vi "GUI_kHz_LPA_backup20250620.vi"() -> ()   [LabVIEW 2020]
uses:
  GUI_TestStand/Fire button.ctl
  Shared/GUI_Template/GUI_master/tcp_new_data_event.ctl
  Shared/GUI_Template/GUI_master/tcp new data cluster.ctl
  Device Drivers/DG645/subVIs/TriggerSource_TypDef.ctl
  <vilib>/Utility/config.llb/Write Key (I32).vi
  <vilib>/Utility/config.llb/NI_LVConfig.lvlib
panel:
  in  "BASE PATH":path=path "Z:/software/control-all-loasis/kHzLPA/Active Version"
  in  "stop":bool
  in  "Tab Control":enum32{"Devices", "Parameters", "Shortcuts"}(tab)=enum."Parameters"
  in  "GUIdevice 6":string="FireContinues"
  in  "GUIdevice 2":string="kHz_1Wire"
  in  "GUIdevice 1":string="kHz_Alicat"
  in  "GUIdevice 3":string="kHz_Hexapod_Target"
  in  "GUIdevice 4":string="kHz_DG645_ShotControl"
  in  "GUIdevice 5":string="kHz_Zaber_Compressor"
  out "error IO":errorcluster
  out "tcp data event":T1
  in  "GUIdevice 7":string="kHz_ESP_TC"
  in  "Scan":T2(ring)
  in  "LogTable":bool
  in  "Mode Imager Button":bool caption="Mode Imager In"
  in  "Step size":dbl=0.01 min=0.001 max=1.0 step=0.001 format="%.3f"
  in  "Rate (Hz)":dbl=0.3
  in  "Fire Continues Checkbox":bool
  out "Fire continues Indicator":bool caption="Fire continuous"
  in  "Trigger.Source::4":T3 caption="SRS Trigger Mode"
  in  "<command>::3":bool caption="ABORT"
  in  "Position.Ch1::5":i32 caption="Ch1" min=0 max=250000 step=1
  in  "Position.Channel 1::2":T4(ring) caption="Fiber Mode"
  in  "Position.Channel 2::2":T4(ring) caption="XH2"
  in  "Position.Channel 3::2":T4(ring) caption="ND6"
  in  "Position.Channel 4::2":T4(ring) caption="XH4"
  in  "Position.Channel 5::2":T4(ring) caption="d-scan wedge"
  in  "Position.Channel 6::2":T4(ring) caption="EC wedge"
  in  "Position.Channel 8::2":T4(ring) caption="Gentec"
  in  "Position.Channel 7::2":T4(ring) caption="Pointing Lanex"
  in  "Pressure.device 1::1":dbl=14.0 caption="Target Pressure" min=0.0 max=100.0
  in  "Pressure.device 2::1":dbl=0.1 caption="Fiber Pressure" min=-14.7 max=500.0
  in  "xpos::3":dbl=-18.95 caption="x" min=-22.5 max=22.5 step=0.009999999999999998 format="%.3f"
  in  "zpos::3":dbl=-0.7 caption="z" min=-10.0 max=10.0 step=0.009999999999999998 format="%.3f"
  in  "ypos::3":dbl=10.7 caption="y" min=-22.5 max=22.5 step=0.009999999999999998 format="%.3f"
  in  "uangle::3":dbl caption="u" min=-7.5 max=7.5 step=0.009999999999999998 format="%.3f"
  in  "vangle::3":dbl=0.0007 caption="v" min=-7.5 max=7.5 step=0.009999999999999998 format="%.3f"
  in  "wangle::3":dbl=-0.0001 caption="w" min=-7.5 max=7.5 step=0.009999999999999998 format="%.3f"
  in  "Fire Button":T5=TRUE
  in  "Jet trigger":bool caption="Jet Trigger"
  in  "Jet enable":bool caption="Jet Enable"
  in  "Set opening time (s)":dbl=0.004
  in  "Amplitude.Ch AB::4":dbl=4.0 caption="Amplitude Jet trigger" min=0.5 max=5.0 format="%.1f"
  in  "Delay.Ch B::4":dbl=0.004 caption="Opening time" min=-0.1 max=0.1 format="%#_6p"
  in  "value0:6":bool caption="Fire continues"
  in  "UDP error message":string
  in  "Position.Axis 2::7":dbl caption="Magent Postition" min=-65.0 max=30.0 format="%.2f"
  in  "Position.Axis 1::7":dbl caption="Mode Imager Position" min=0.0 max=25.0 format="%.2f"
  in  "fire::4":string="fire>>force" caption="fire text"
  in  "Position.Axis 3::7":dbl caption="Probe Delay" min=0.0 max=25.0 format="%.2f"
  in  "Create Log":bool caption="LogTable"
  in  "LogEpilog":bool caption="LogTable"
  in  "Gen new log?":bool
  in  "Search Log":bool caption="PicoL GUI"
  in  "RemoteDesktop":bool caption="PicoL GUI"
  in  "kHz Interactive":bool caption="PicoL GUI"
  in  "Exp Editor":bool caption="PicoL GUI"
  in  "DB Editor":bool caption="PicoL GUI"
  in  "AddColumns":bool caption="PicoL GUI"
  in  "GEECSplot":bool caption="PicoL GUI"
  in  "MasterControl":bool caption="PicoL GUI"
  in  "Google Drive":bool
  in  "LVStarter":bool caption="PicoL GUI"
  out "standard output":string="04-16-21\r\n04-16-21 kHz Scanlog\r\nZ:/data/kHzLPA/Y2021/04-Apr/21_0416/scans\\Scan001\r\nSearch updated: 04-16-21.*Scan 1:\r\n**Establish Server Connection with Google Cloud**\r\n...Service created successfully\r\n<googleapiclient.discovery.Resource object at 0x000001F266DE75B0>\r\n**Append template to document...**\r\n... success\r\n**Scanfiles found**\r\nZ:/data/kHzLPA/Y2021/04-Apr/21_0416/ECS Live dumps\\Scan1.txt\r\nZ:/data/kHzLPA/Y2021/04-Apr/21_0416/scans\\Scan001\\ScanInfoScan001.ini\r\n**Find and replace placeholders with current values**\r\n**Establish Server Connection with Google Cloud**\r\n...Service created successfully\r\n<googleapiclient.discovery.Resource object at 0x000001F266EB5790>\r\n**Adding screenshot**\r\n"
  # "kHz control center"
  # "Laser"
  # "1-wire flippers"
  # "\"+x\" is towards laser table\n\"+y\" is towards OAP\n\"+z\" is up"
  # "ABORT !"
  # "Tobi's LogMaker"
  # "Compressor"
  # "Alicat"
  # "New\nScan\nTable"
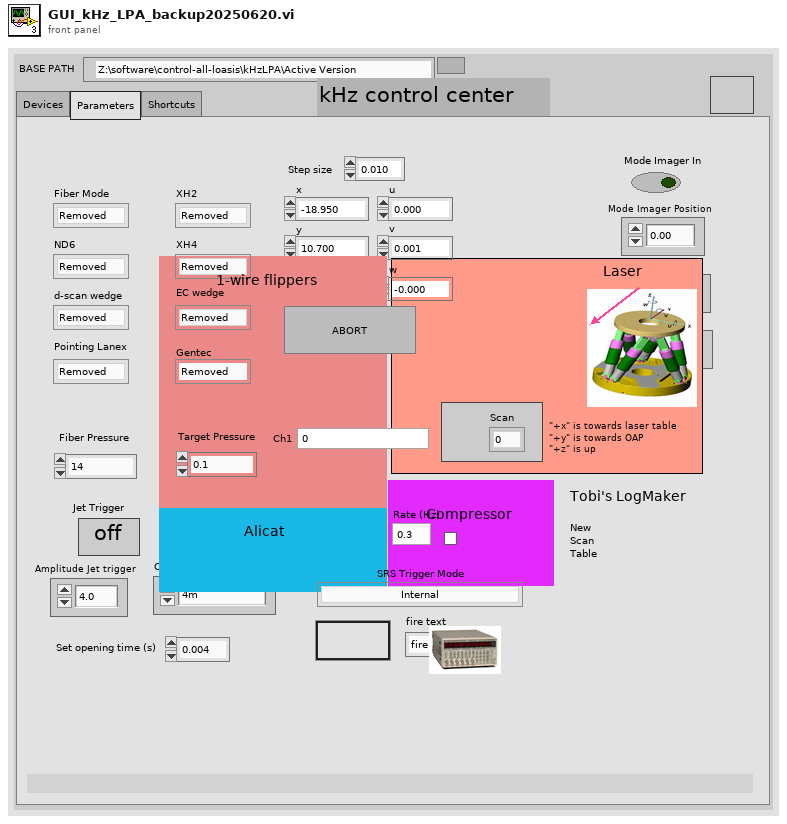
[diagram p1: front panel]
types:
  T1 = typedef "tcp_new_data_event.ctl" = refnum<user-event>
  T2 = enum16{"0", "1", "2", "3", "4", "5", "6", "7", "8", "9", "10", "11", "12", "13", "14", "15", "16", "17", "18", "19", "20", "21", "22", "23", "24", "25", "26", "27", "28", "29", "30", "31", "32", "33", "34", "35", "36", "37", "38", "39", "40", "41", "42", "43", "44", "45", "46", "47", "48", "49", "50", "51", "52", "53", "54", "55", "56", "57", "58", "59", "60", "61", "62", "63", "64", "65", "66", "67", "68", "69", "70", "71", "72", "73", "74", "75", "76", "77", "78", "79", "81", "82", "83", "84", "85", "86", "87", "88", "89", "90", "91", "92", "93", "94", "95", "96", "97", "98", "99", ""}
  T3 = typedef "TriggerSource_TypDef.ctl" = enum16{"Internal", "External rising edges", "External falling edges", "Single shot external rising edges", "Single shot external falling edges", "Single shot", "Line"}
  T4 = enum16{"Removed", "Inserted", "Unknown", "Moving"}
  T5 = typedef "Fire button.ctl" = bool
  T6 = typedef "tcp new data cluster.ctl" = cluster{"EventEnum":enum16{"new data", "connection status update"}, "Device name":string}
  T7 = enum32{"Invalid", "Standard", "Closed", "Hidden", "Minimized", "Maximized"}
  T8 = enum32{"invalid app kind", "Development System", "Run Time System", "Student Edition", "Embedded LabVIEW", "Evaluation", "Custom"}
  T9 = cluster{"Core":cluster{"Current VI Reference":refnum<vi>, "Close Panel on Exit?":bool}, "Jet enable":bool, "Jet trigger":bool, "Fire Continues Allowed":bool, "Tik1":u32, "ModeImagerIn":bool}
  T10 = typedef "imagedata.ctl" = cluster{"image type":i32, "image depth":i32, "image":u8[], "mask":u8[], "colors":u32[], "Rectangle":cluster{"left":i16, "top":i16, "right":i16, "bottom":i16}}
  T11 = typedef "NI_LVConfig.lvlib/Config Data RefNum.ctl" = refnum<k1>
  T12 = cluster{"Current VI Reference":refnum<vi>, "Close Panel on Exit?":bool}
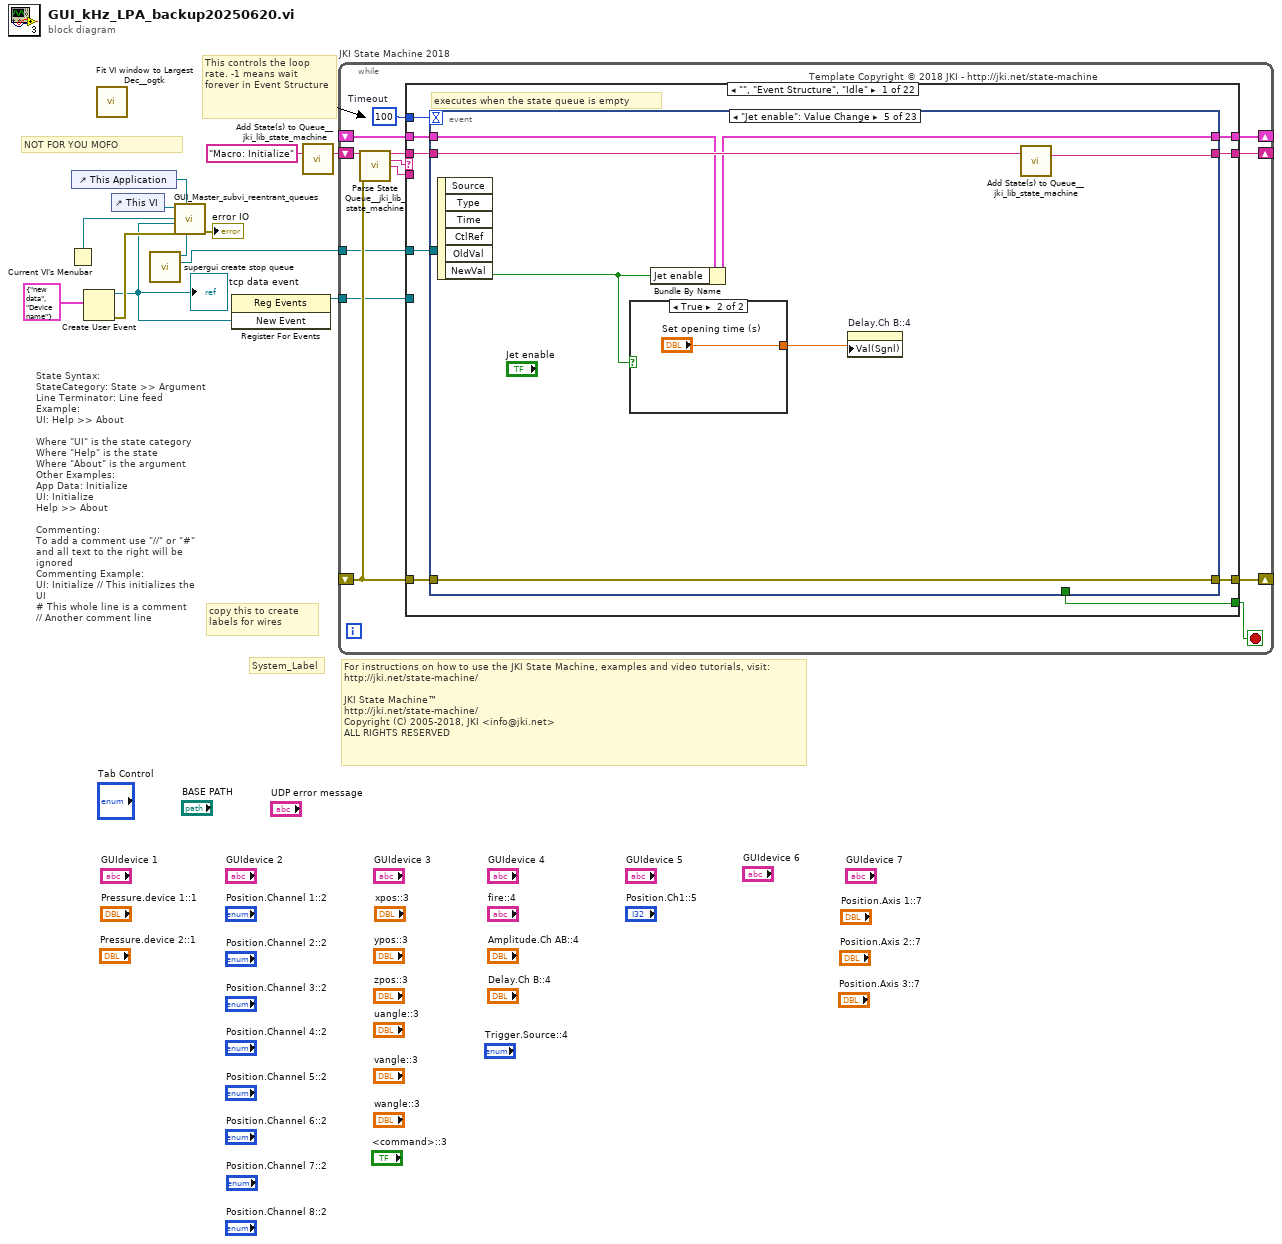
[diagram p0: block diagram]
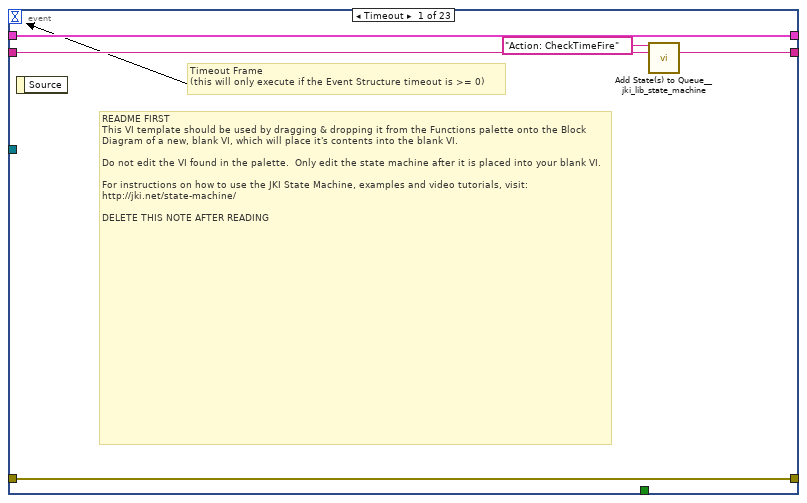
[diagram p2: hidden frame]
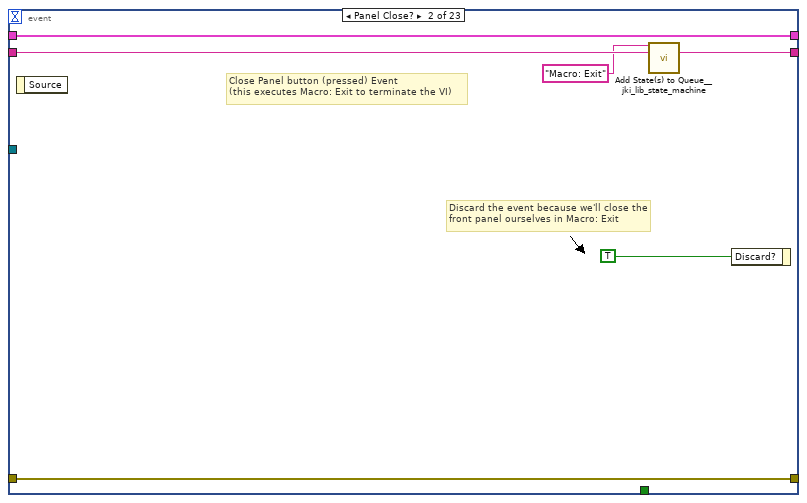
[diagram p3: hidden frame]
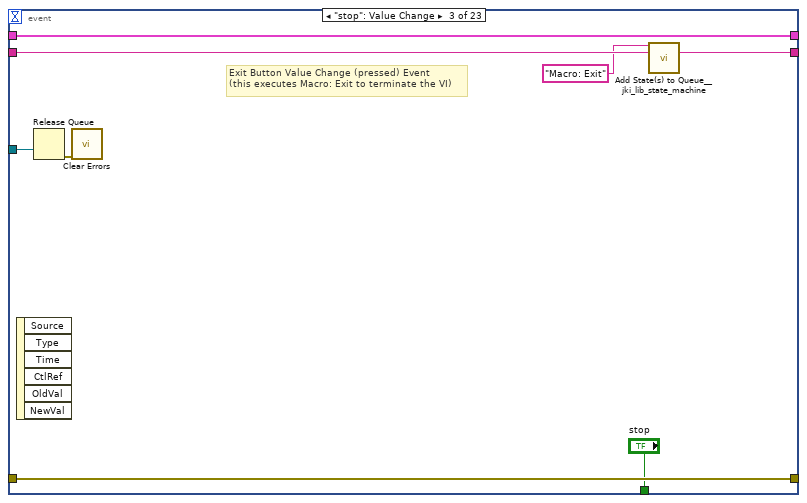
[diagram p4: hidden frame]
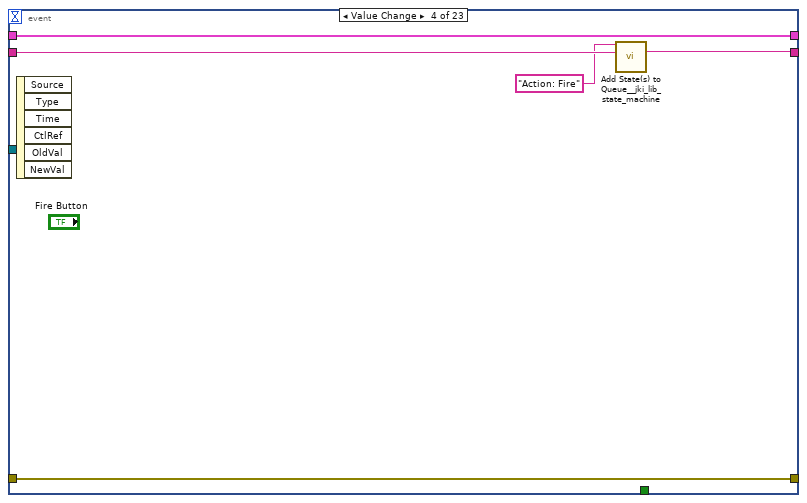
[diagram p5: hidden frame]
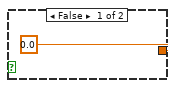
[diagram p6: hidden frame]
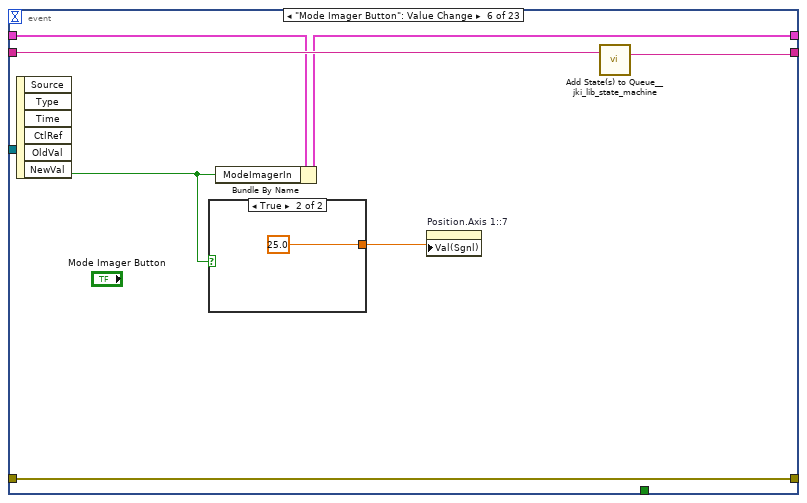
[diagram p7: hidden frame]
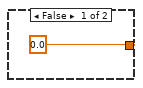
[diagram p8: hidden frame]
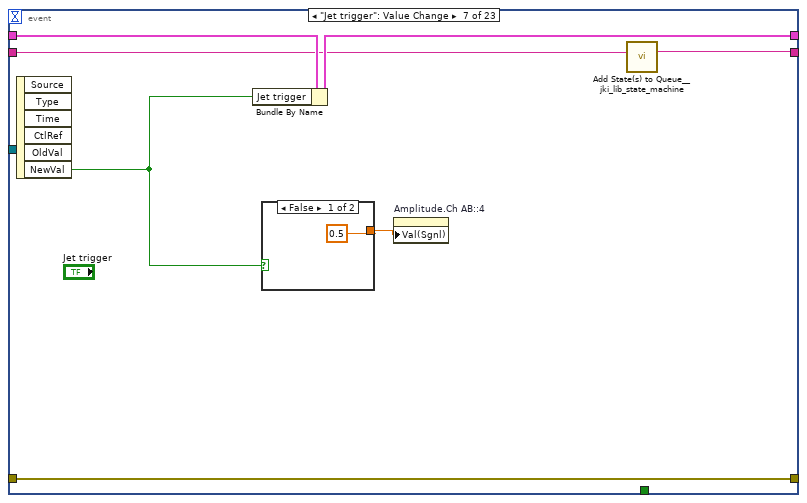
[diagram p9: hidden frame]
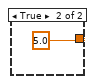
[diagram p10: hidden frame]
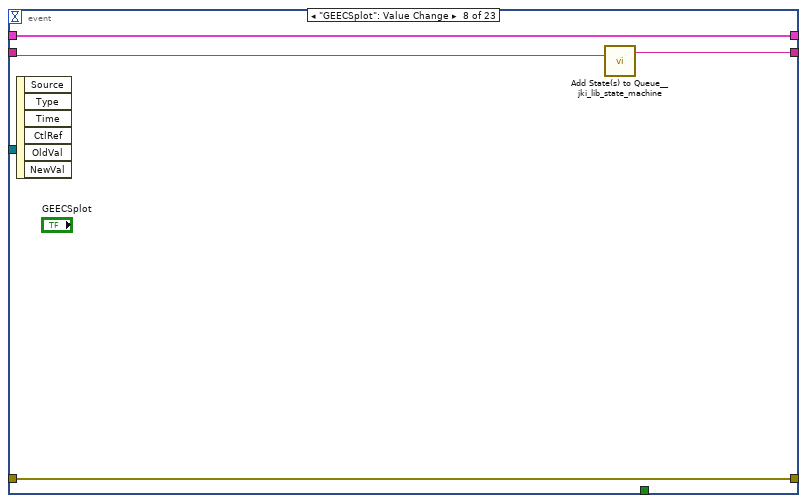
[diagram p11: hidden frame]
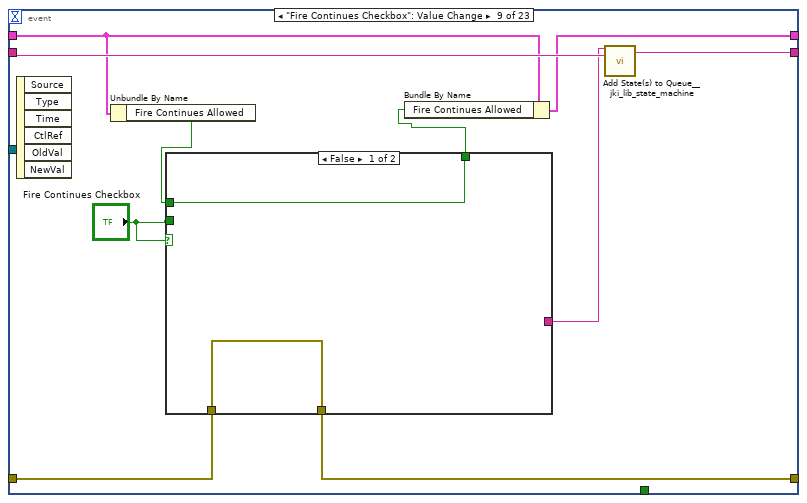
[diagram p12: hidden frame]
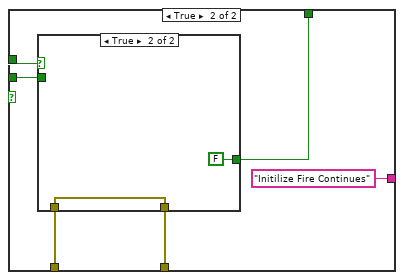
[diagram p13: hidden frame]
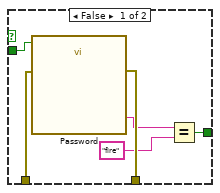
[diagram p14: hidden frame]
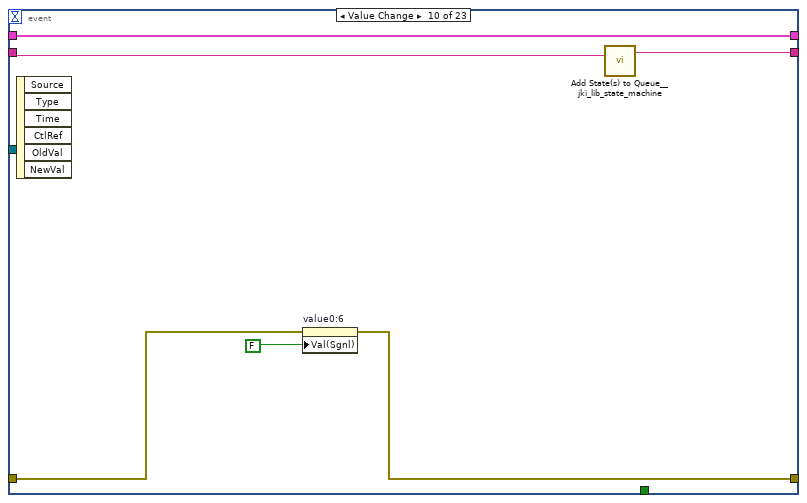
[diagram p15: hidden frame]
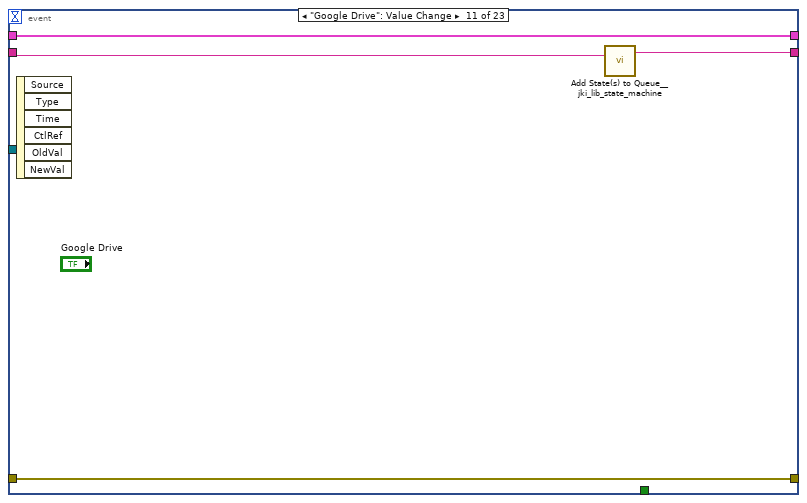
[diagram p16: hidden frame]
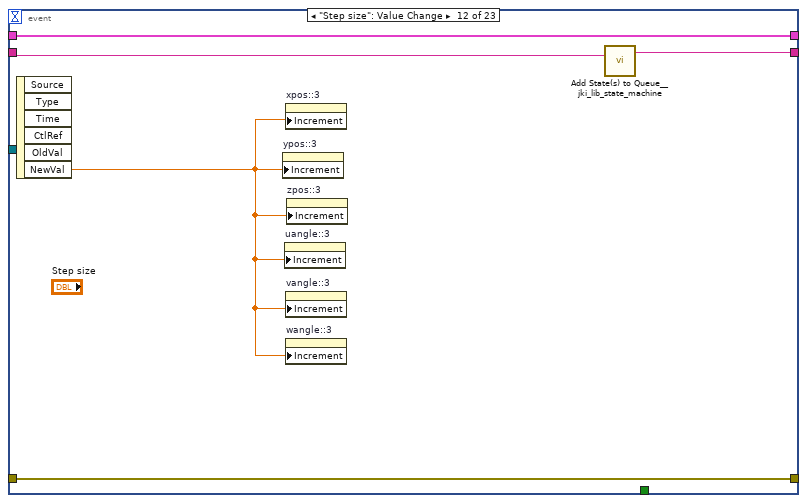
[diagram p17: hidden frame]
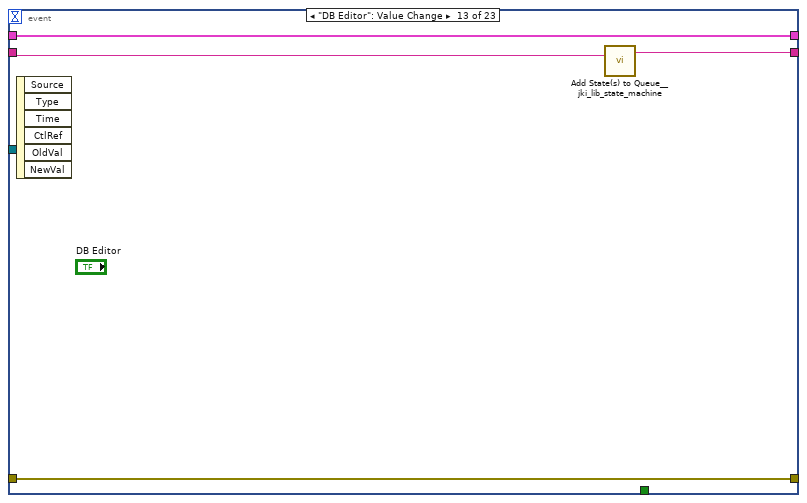
[diagram p18: hidden frame]
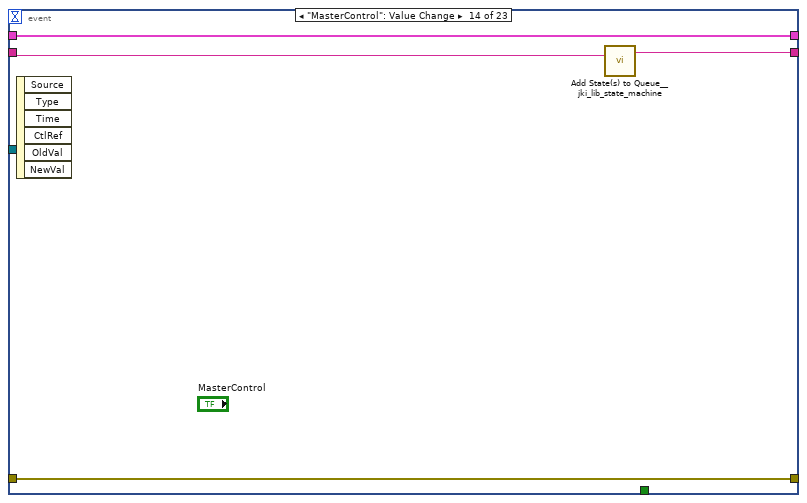
[diagram p19: hidden frame]
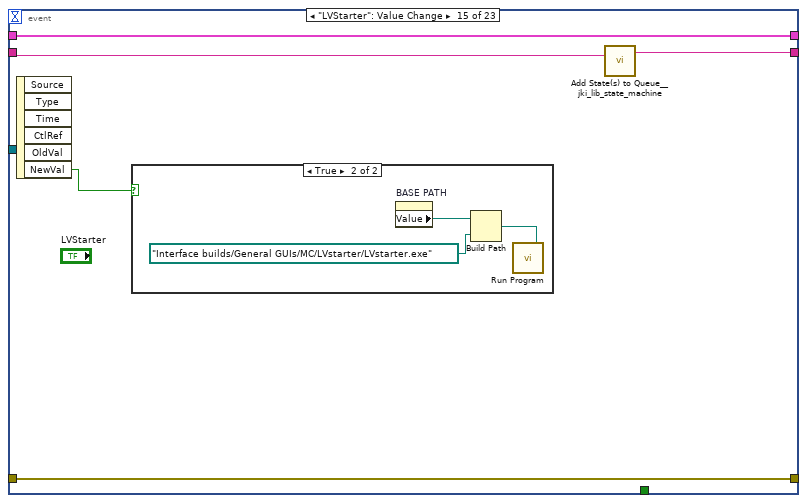
[diagram p20: hidden frame]
diagram:
  # "NOT FOR YOU MOFO"
  # "For instructions on how to use the JKI State Machine, examples and video tutorials, visit:\nhttp://jki.net/state-machine/\n\nJKI State Machine™\nhttp://jki.net/state-machine/\nCopyright (C) 2005-2018, JKI <info@jki.net>\nALL RIGHTS RESERVED"
  # "State Syntax:\nStateCategory: State >> Argument\nLine Terminator: Line feed\nExample:\nUI: Help >> About\n\nWhere \"UI\" is the state category\nWhere \"Help\" is the state\nWhere \"About\" is the argument\nOther Examples:\nApp Data: Initialize\nUI: Initialize\nHelp >> About\n\nCommenting:\nTo add a comment use \"//\" or \"#\" and all text to the right will be ignored\nCommenting Example:\nUI: Initialize // This initializes the UI\n# This whole line is a comment\n// Another comment line"
  # "copy this to create labels for wires"
  # "This controls the loop rate. -1 means wait forever in Event Structure"
  # "System_Label"
  n1 = Current VI's Menubar() -> (w6:refnum<k9>)
  n2 = control-ref of="This Application"() -> (w9:refnum<vi>)
  n3 = Create User Event(user event datatype=T6 {"EventEnum"=enum."new data", "Device name"="Device name"} ("New Event")) -> (user event=w3:refnum<user-event>, error out=w8:errorcluster)  [unwired: 1 in]
  "tcp data event" <- w3
  n4 = call <userlib>:"Fit VI window to Largest Dec__ogtk.vi"() -> ()  [unwired: 6 in, 2 out]
  n5 = control-ref of="This VI"() -> (w5:refnum<vi>)
  n6 = call "supergui create stop queue.vi"() -> ("STOP Queue out"=w2:refnum<queue>)  [unwired: 11 in]
  n7 = call "GUI_Master_subvi_reentrant_queues.vi"("STOP Queue in"=w2, "This Application"=w9, "error in (no error)"=w8, "tcp data event"=w3, "Caller menu reference"=w6, "Caller VI ref"=w5) -> ("error out"=→"error IO":errorcluster)  [unwired: 5 in]
  n8 = register-events(w3) -> (reference out=w1:refnum<event-registration>)  [unwired: 2 in, 1 out]
  n9 = call <vilib>:"Add State(s) to Queue__jki_lib_state_machine.vi"("State(s) in (\"\")"="Macro: Initialize") -> ("States Out"=w11:string)  [unwired: 14 in]
  n10 = while "JKI State Machine 2018" {
    shift-right: [w17] -> _
    shift-left: _ -> [w16]
    shift-right: [w20] -> _
    shift-left: _ -> [w14]
    shift-right: [w19] -> _
    shift-left: w11 -> [w21]
    tunnel: w2 -> [w13]
    tunnel: w1 -> [w12]
    stop <- w18 stop-if-true
    w15 = 100  # Timeout
    # "Template Copyright © 2018 JKI - http://jki.net/state-machine"
    n11 = call <vilib>:"Parse State Queue__jki_lib_state_machine.vi"("State Queue"=w21, "Error In (no error)"=w14) -> ("Remaining States"=w23:string, "Current State"=w24:string, "Arguments"=w22:string)  [unwired: 11 in]
    n12 = case shown="\"\", \"Event Structure\", \"Idle\"" w24 {
      selector: w24 -> [_ _ w257 _ _ _ _ _ _ _ _ _ _ _ _ _ _ _ _ _ _ _]
      tunnel: w23 -> [w33 w256 w261 w280 w286 w291 w295 w305 w311 w315 w319 w325 w336 w405 w410 w420 w424 w430 w434 w442 w454 w473]
      tunnel: w22 -> [_ _ _ _ _ _ _ _ _ _ _ w320 w330 _ _ _ _ _ _ _ _ _]
      tunnel: w16 -> [w31 w253 w259 w273 w283 w289 w292 _ w306 w312 w317 w323 w332 w402 w407 w417 w421 w428 w432 w437 w446 w458]
      tunnel: [w30 w254 w263 w277 errorcluster {"status"=FALSE, "code"=0, "source"=""} ("error out") w288 w293 w302 w307 w313 w316 w321 w333 w403 w408 w418 w422 w425 w431 w435 w444 w471] -> w20
      tunnel: w14 -> [w29 w254 w262 w277 w282 w288 w293 w302 w308 w313 w316 w322 w334 w403 w408 w418 w422 w426 w431 w436 w443 w471]
      tunnel: [w32 w255 w260 w279 w285 w290 w294 w304 w310 w314 w318 w324 w335 w404 w409 w419 w423 w429 w433 w441 w453 w472] -> w19
      tunnel: [w25 _ _ _ _ TRUE _ _ _ _ _ _ _ _ _ _ _ _ _ _ _ _] -> w18
      tunnel: [w28 w253 w259 w278 w283 w289 w292 w303 w306 w312 w317 w323 w332 w402 w407 w417 w421 w428 w432 w437 w445 w457] -> w17
      tunnel: w15 -> [w27 _ _ _ _ _ _ _ _ _ _ _ _ _ _ _ _ _ _ _ _ _]
      tunnel: w13 -> [w26 _ _ _ _ _ _ _ _ _ _ _ _ _ _ _ _ _ _ _ _ _]
      tunnel: w12 -> [_ _ _ _ _ _ _ _ _ _ _ _ _ _ _ _ _ _ _ _ _ _]
      frame "", "Event Structure", "Idle" {
        # "executes when the state queue is empty"
        n13 = event shown="[4] \"Jet enable\": Value Change" {
          selector: _ -> [_ _ _ _ _ _ _ _ _ _ _ _ _ _ _ _ _ _ _ _ _ _ _]
          dyn-events: _ -> [_ _ _ _ _ _ _ _ _ _ _ _ _ _ _ _ _ _ _ _ _ _ _]
          timeout: w27 -> [_ _ _ _ _ _ _ _ _ _ _ _ _ _ _ _ _ _ _ _ _ _ _]
          tunnel: w33 -> [w38 w44 w52 w56 w62 w71 w76 w86 w97 w118 w122 w127 w131 w135 w139 w149 w153 w155 w160 w189 w228 w232 w237]
          tunnel: [w37 w43 w51 w57 w63 w72 w77 w87 w98 w119 w123 w128 w132 w136 w140 w148 w152 w156 w161 w190 w229 w233 w238] -> w32
          tunnel: w31 -> [w35 w41 w49 w55 w61 w70 w81 w88 w96 w120 w124 w129 w133 w137 w141 w146 w150 w154 w159 w188 w227 w231 w236]
          tunnel: [w36 w42 w50 w53 w58 w67 w78 w85 w89 w115 w121 w126 w130 w134 w138 w147 w151 w157 w162 w191 w230 w234 w239] -> w30
          tunnel: w29 -> [w36 w42 w50 w53 w58 w67 w78 w85 w90 w116 w121 w126 w130 w134 w138 w147 w151 w157 w162 w191 w230 w234 w239]
          tunnel: [w35 w41 w49 w55 w60 w69 w79 w88 w95 w120 w124 w129 w133 w137 w141 w146 w150 w154 w159 w188 w227 w231 w236] -> w28
          tunnel: w26 -> [_ _ w46 _ _ _ _ _ _ _ _ _ _ _ _ _ _ _ _ _ _ _ _]
          tunnel: [_ _ "stop" _ _ _ _ _ _ _ _ _ _ _ _ _ _ _ _ _ _ _ _] -> w25
          event Timeout {
            # "README FIRST\nThis VI template should be used by dragging & dropping it from the Functions palette onto the Block Diagram of a new, blank VI, which will place it's contents into the blank VI.\n\nDo not edit the VI found in the palette.  Only edit the state machine after it is placed into your blank VI.\n\nFor instructions on how to use the JKI State Machine, examples and video tutorials, visit:\nhttp://jki.net/state-machine/\n\nDELETE THIS NOTE AFTER READING"
            # "Timeout Frame\n(this will only execute if the Event Structure timeout is >= 0)"
            n14 = event-data() -> ()  [unwired: 1 in, 1 out]
            n15 = call <vilib>:"Add State(s) to Queue__jki_lib_state_machine.vi"("State(s) in Front (\"\")"="Action: CheckTimeFire" ("State(s) in Front (\"\")"), "State(s) in (\"\")"=w38) -> ("States Out"=w37:string)  [unwired: 13 in]
          }
          event Panel Close? {
            # "Discard the event because we'll close the front panel ourselves in Macro: Exit"
            # "Close Panel button (pressed) Event\n(this executes Macro: Exit to terminate the VI)"
            n16 = event-data() -> ()  [unwired: 1 in, 1 out]
            n17 = call <vilib>:"Add State(s) to Queue__jki_lib_state_machine.vi"("State(s) in Front (\"\")"="Macro: Exit", "State(s) in (\"\")"=w44) -> ("States Out"=w43:string)  [unwired: 13 in]
            n18 = event-data("Discard?"=TRUE) -> ()  [unwired: 1 in, 1 out]
          }
          event "stop": Value Change {
            # "Exit Button Value Change (pressed) Event\n(this executes Macro: Exit to terminate the VI)"
            n19 = event-data() -> ()  [unwired: 1 in, 6 out]
            n20 = Release Queue(queue=w46) -> (error out=w47:errorcluster)  [unwired: 2 in, 2 out]
            n21 = call <vilib>:"Clear Errors.vi"("error in (no error)"=w47) -> ()  [unwired: 5 in, 2 out]
            n22 = call <vilib>:"Add State(s) to Queue__jki_lib_state_machine.vi"("State(s) in Front (\"\")"="Macro: Exit", "State(s) in (\"\")"=w52) -> ("States Out"=w51:string)  [unwired: 13 in]
          }
          event Value Change {
            n23 = event-data() -> ()  [unwired: 1 in, 6 out]
            n24 = call <vilib>:"Add State(s) to Queue__jki_lib_state_machine.vi"("State(s) in Front (\"\")"="Action: Fire" ("State(s) in Front (\"\")"), "State(s) in (\"\")"=w56) -> ("States Out"=w57:string)  [unwired: 13 in]
          }
          event "Jet enable": Value Change {
            n25 = event-data() -> ("NewVal"=w59:bool)  [unwired: 1 in, 5 out]
            n26 = case shown="True" w59 {
              tunnel: [0.0 ("opening Time") "Set opening time (s)"] -> w64
              frame False {
              }
              frame True {
              }
            }
            n27 = Bundle By Name(cluster=w61, "Jet enable"=w59) -> (w60:T9)
            n28 = property on="Delay.Ch B::4" class="DigNum (strict)"("Val(Sgnl)"=w64) -> ()  [unwired: 2 in, 2 out]
            n29 = call <vilib>:"Add State(s) to Queue__jki_lib_state_machine.vi"("State(s) in (\"\")"=w62) -> ("States Out"=w63:string)  [unwired: 14 in]
          }
          event "Mode Imager Button": Value Change {
            n30 = event-data() -> ("NewVal"=w68:bool)  [unwired: 1 in, 5 out]
            n31 = case shown="True" w68 {
              tunnel: [0.0 ("opening Time") 25.0] -> w73
              frame False {
              }
              frame True {
              }
            }
            n32 = Bundle By Name(cluster=w70, "ModeImagerIn"=w68) -> (w69:T9)
            n33 = property on="Position.Axis 1::7" class="DigNum (strict)"("Val(Sgnl)"=w73) -> ()  [unwired: 2 in, 2 out]
            n34 = call <vilib>:"Add State(s) to Queue__jki_lib_state_machine.vi"("State(s) in (\"\")"=w71) -> ("States Out"=w72:string)  [unwired: 14 in]
          }
          event "Jet trigger": Value Change {
            n35 = event-data() -> ("NewVal"=w80:bool)  [unwired: 1 in, 5 out]
            n36 = Bundle By Name(cluster=w81, "Jet trigger"=w80) -> (w79:T9)
            n37 = case shown="False" w80 {
              tunnel: [0.5 ("Amplitude.Ch CD::10") 5.0 ("Amplitude.Ch CD::10")] -> w82
              frame False {
              }
              frame True {
              }
            }
            n38 = property on="Amplitude.Ch AB::4" class="DigNum (strict)"("Val(Sgnl)"=w82) -> ()  [unwired: 2 in, 2 out]
            n39 = call <vilib>:"Add State(s) to Queue__jki_lib_state_machine.vi"("State(s) in (\"\")"=w76) -> ("States Out"=w77:string)  [unwired: 14 in]
          }
          event "GEECSplot": Value Change {
            n40 = event-data() -> ()  [unwired: 1 in, 6 out]
            n41 = call <vilib>:"Add State(s) to Queue__jki_lib_state_machine.vi"("State(s) in (\"\")"=w86) -> ("States Out"=w87:string)  [unwired: 14 in]
          }
          event "Fire Continues Checkbox": Value Change {
            n42 = event-data() -> ()  [unwired: 1 in, 6 out]
            n43 = Unbundle By Name(w96) -> ("Fire Continues Allowed"=w91:bool)
            n44 = case shown="False" "Fire Continues Checkbox" {
              tunnel: [w99 w106] -> w89
              tunnel: "Fire Continues Checkbox" -> [_ w105]
              tunnel: w90 -> [w99 w104]
              tunnel: w91 -> [w100 w103]
              tunnel: [w100 w101] -> w93
              tunnel: [_ "Initilize Fire Continues" ("State(s) in Front (\"\")")] -> w94
              frame False {
              }
              frame True {
                n45 = case shown="True" w103 {
                  tunnel: [w112 w113] -> w106
                  tunnel: w105 -> [w111 _]
                  tunnel: w104 -> [w110 w113]
                  tunnel: [w107 FALSE] -> w101
                  frame False {
                    n46 = call "Password"("Enable"=w111, "error in (no error)"=w110) -> ("Password"=w109:string, "error out"=w112:errorcluster)  [unwired: 15 in, 1 out]
                    n47 = Equal?(x=w109, y="fire") -> (x = y?=w107:bool)
                  }
                  frame True {
                  }
                }
              }
            }
            n48 = Bundle By Name(cluster=w96, "Fire Continues Allowed"=w93) -> (w95:T9)
            n49 = call <vilib>:"Add State(s) to Queue__jki_lib_state_machine.vi"("State(s) in Front (\"\")"=w94, "State(s) in (\"\")"=w97) -> ("States Out"=w98:string)  [unwired: 13 in]
          }
          event Value Change {
            n50 = event-data() -> ()  [unwired: 1 in, 6 out]
            n51 = property on="value0:6" class="Bool (strict)"(error in=w116, "Val(Sgnl)"=FALSE) -> (error out=w115:errorcluster)  [unwired: 1 in, 1 out]
            n52 = call <vilib>:"Add State(s) to Queue__jki_lib_state_machine.vi"("State(s) in (\"\")"=w118) -> ("States Out"=w119:string)  [unwired: 14 in]
          }
          event "Google Drive": Value Change {
            n53 = event-data() -> ()  [unwired: 1 in, 6 out]
            n54 = call <vilib>:"Add State(s) to Queue__jki_lib_state_machine.vi"("State(s) in (\"\")"=w122) -> ("States Out"=w123:string)  [unwired: 14 in]
          }
          event "Step size": Value Change {
            n55 = event-data() -> ("NewVal"=w125:dbl)  [unwired: 1 in, 5 out]
            n56 = property on="ypos::3" class="DigNum (strict)"("Increment"=w125) -> ()  [unwired: 2 in, 2 out]
            n57 = property on="uangle::3" class="DigNum (strict)"("Increment"=w125) -> ()  [unwired: 2 in, 2 out]
            n58 = property on="xpos::3" class="DigNum (strict)"("Increment"=w125) -> ()  [unwired: 2 in, 2 out]
            n59 = property on="vangle::3" class="DigNum (strict)"("Increment"=w125) -> ()  [unwired: 2 in, 2 out]
            n60 = property on="wangle::3" class="DigNum (strict)"("Increment"=w125) -> ()  [unwired: 2 in, 2 out]
            n61 = property on="zpos::3" class="DigNum (strict)"("Increment"=w125) -> ()  [unwired: 2 in, 2 out]
            n62 = call <vilib>:"Add State(s) to Queue__jki_lib_state_machine.vi"("State(s) in (\"\")"=w127) -> ("States Out"=w128:string)  [unwired: 14 in]
          }
          event "DB Editor": Value Change {
            n63 = event-data() -> ()  [unwired: 1 in, 6 out]
            n64 = call <vilib>:"Add State(s) to Queue__jki_lib_state_machine.vi"("State(s) in (\"\")"=w131) -> ("States Out"=w132:string)  [unwired: 14 in]
          }
          event "MasterControl": Value Change {
            n65 = event-data() -> ()  [unwired: 1 in, 6 out]
            n66 = call <vilib>:"Add State(s) to Queue__jki_lib_state_machine.vi"("State(s) in (\"\")"=w135) -> ("States Out"=w136:string)  [unwired: 14 in]
          }
          event "LVStarter": Value Change {
            n67 = event-data() -> ("NewVal"=w142:bool)  [unwired: 1 in, 5 out]
            n68 = case shown="True" w142 {
              frame False {
              }
              frame True {
                n69 = property on="BASE PATH" class="Path"() -> ("Value"=w143:path)  [unwired: 2 in, 2 out]
                n70 = Build Path(base path=w143, name or relative path=path "Interface builds/General GUIs/MC/LVstarter/LVstarter.exe") -> (appended path=w145:path)
                n71 = call "Run Program.vi"("Program Path"=w145) -> ()  [unwired: 1 in]
              }
            }
            n72 = call <vilib>:"Add State(s) to Queue__jki_lib_state_machine.vi"("State(s) in (\"\")"=w139) -> ("States Out"=w140:string)  [unwired: 14 in]
          }
          event "kHz Interactive": Value Change {
            n73 = event-data() -> ()  [unwired: 1 in, 6 out]
            n74 = call <vilib>:"Add State(s) to Queue__jki_lib_state_machine.vi"("State(s) in (\"\")"=w149) -> ("States Out"=w148:string)  [unwired: 14 in]
          }
          event "RemoteDesktop": Value Change {
            n75 = event-data() -> ()  [unwired: 1 in, 6 out]
            n76 = call <vilib>:"Add State(s) to Queue__jki_lib_state_machine.vi"("State(s) in (\"\")"=w153) -> ("States Out"=w152:string)  [unwired: 14 in]
          }
          event "Exp Editor": Value Change {
            n77 = event-data() -> ()  [unwired: 1 in, 6 out]
            n78 = call <vilib>:"Add State(s) to Queue__jki_lib_state_machine.vi"("State(s) in (\"\")"=w155) -> ("States Out"=w156:string)  [unwired: 14 in]
          }
          event "LogEpilog": Value Change {
            n79 = event-data() -> ("NewVal"=w158:bool)  [unwired: 1 in, 5 out]
            n80 = case shown="True" w158 {
              frame False {
              }
              frame True {
                n81 = call <vilib>:"Space Constant.vi"() -> ("String"=w169:string)
                n82 = call <vilib>:"Space Constant.vi"() -> ("String"=w167:string)
                n83 = call <vilib>:"Space Constant.vi"() -> ("String"=w165:string)
                n84 = Concatenate Strings("cmd /c python appendEpilog.py", w169, "KHZparameters.ini", w167, "KHZplaceholders.ini", w165, "KHZcurrentvalues.ini") -> (w163:string)
                n85 = property on="BASE PATH" class="Path"() -> ("Value"=w173:path)  [unwired: 2 in, 2 out]
                n86 = Build Path(base path=w173, name or relative path=path "GEECS-Plugins/LogMaker 4 GoogleDocs/source" ("working directory")) -> (appended path=w172:path)
                n87 = call <vilib>:"System Exec.vi"("expected output size  (4096)"=u32 1000000, "run minimized? (F)"=FALSE, "working directory"=w172, "command line"=w163) -> ()  [unwired: 4 in, 4 out]
              }
            }
            n88 = call <vilib>:"Add State(s) to Queue__jki_lib_state_machine.vi"("State(s) in (\"\")"=w160) -> ("States Out"=w161:string)  [unwired: 14 in]
          }
          event "LogTable": Value Change {
            n89 = event-data() -> ("NewVal"=w187:bool)  [unwired: 1 in, 5 out]
            n90 = case shown="True" w187 {
              frame False {
              }
              frame True {
                n91 = flat-sequence {
                  frame #0 {
                    n92 = invoke class="VI" method="FP.Get Image"() -> ("image data"=w195:T10)  [unwired: 6 in, 5 out]
                    n93 = property on="BASE PATH" class="Path"() -> ("Value"=w194:path)  [unwired: 2 in, 2 out]
                    n94 = Build Path(base path=w194, name or relative path=path "GEECS-Plugins/LogMaker 4 GoogleDocs/source/frontpanel.png" ("report file path")) -> (appended path=w193:path)
                    n95 = call <vilib>:"Write PNG File.vi"("image data"=w195, "path to PNG file"=w193) -> ()  [unwired: 8 in, 2 out]
                  }
                  frame #1 {
                    n96 = Wait (ms)(milliseconds to wait=u32 200 ("millisecond timer value")) -> ()  [unwired: 1 out]
                  }
                  frame #2 {
                    n97 = case shown="True" "Gen new log?" {
                      tunnel: [w210 w224] -> w198
                      frame False {
                        n98 = call <vilib>:"Space Constant.vi"() -> ("String"=w205:string)
                        n99 = call <vilib>:"Space Constant.vi"() -> ("String"=w203:string)
                        n100 = call <vilib>:"Space Constant.vi"() -> ("String"=w201:string)
                        n101 = Concatenate Strings("cmd /c python appendScanOldLog.py", w205, "KHZparameters.ini", w203, "KHZplaceholders.ini", w201, "KHZcurrentvalues.ini") -> (w199:string)
                        n102 = property on="BASE PATH" class="Path"() -> ("Value"=w209:path)  [unwired: 2 in, 2 out]
                        n103 = Build Path(base path=w209, name or relative path=path "GEECS-Plugins/LogMaker 4 GoogleDocs/source" ("working directory")) -> (appended path=w208:path)
                        n104 = call <vilib>:"System Exec.vi"("expected output size  (4096)"=u32 1000000, "run minimized? (F)"=FALSE, "working directory"=w208, "command line"=w199) -> ("standard output"=w210:string)  [unwired: 4 in, 3 out]
                      }
                      frame True {
                        n105 = call <vilib>:"Space Constant.vi"() -> ("String"=w219:string)
                        n106 = call <vilib>:"Space Constant.vi"() -> ("String"=w217:string)
                        n107 = call <vilib>:"Space Constant.vi"() -> ("String"=w215:string)
                        n108 = Concatenate Strings("cmd /c python appendScan.py", w219, "KHZparameters.ini", w217, "KHZplaceholders.ini", w215, "KHZcurrentvalues.ini") -> (w213:string)
                        n109 = property on="BASE PATH" class="Path"() -> ("Value"=w223:path)  [unwired: 2 in, 2 out]
                        n110 = Build Path(base path=w223, name or relative path=path "GEECS-Plugins/LogMaker 4 GoogleDocs/source" ("working directory")) -> (appended path=w222:path)
                        n111 = call <vilib>:"System Exec.vi"("expected output size  (4096)"=u32 1000000, "run minimized? (F)"=FALSE, "working directory"=w222, "command line"=w213) -> ("standard output"=w224:string)  [unwired: 4 in, 3 out]
                      }
                    }
                    "standard output" <- w198
                  }
                }
              }
            }
            n112 = property on="BASE PATH" class="Path"() -> ("Value"=w185:path)  [unwired: 2 in, 2 out]
            n113 = Build Path(base path=w185, name or relative path=path "GEECS-Plugins/LogMaker 4 GoogleDocs/source/KHZparameters.ini") -> (appended path=w186:path)
            n114 = call <vilib>:"Open Config Data.vi"("configuration file path"=w186) -> ("error out"=w183:errorcluster, "refnum"=w181:T11)  [unwired: 8 in, 1 out]
            n115 = call-poly <vilib>:"Write Key.vi"("section"="SCAN", "error in (no error)"=w183, "value"="Scan", "key"="scannumber", "refnum"=w181) -> ("error out"=w184:errorcluster, "refnum out"=w182:T11)  [unwired: 4 in, 1 out]
            n116 = call <vilib>:"Add State(s) to Queue__jki_lib_state_machine.vi"("State(s) in (\"\")"=w189) -> ("States Out"=w190:string)  [unwired: 14 in]
            n117 = call <vilib>:"Close Config Data.vi"("error in (no error)"=w184, "write file if changed (T)"=TRUE, "refnum"=w182) -> ()  [unwired: 7 in, 2 out]
          }
          event "Search Log": Value Change {
            n118 = event-data() -> ()  [unwired: 1 in, 6 out]
            n119 = call <vilib>:"Add State(s) to Queue__jki_lib_state_machine.vi"("State(s) in (\"\")"=w228) -> ("States Out"=w229:string)  [unwired: 14 in]
          }
          event "AddColumns": Value Change {
            n120 = event-data() -> ()  [unwired: 1 in, 6 out]
            n121 = call <vilib>:"Add State(s) to Queue__jki_lib_state_machine.vi"("State(s) in (\"\")"=w232) -> ("States Out"=w233:string)  [unwired: 14 in]
          }
          event "Create Log": Value Change {
            n122 = event-data() -> ("NewVal"=w235:bool)  [unwired: 1 in, 5 out]
            n123 = case shown="True" w235 {
              frame False {
              }
              frame True {
                n124 = call <vilib>:"Space Constant.vi"() -> ("String"=w246:string)
                n125 = call <vilib>:"Space Constant.vi"() -> ("String"=w244:string)
                n126 = call <vilib>:"Space Constant.vi"() -> ("String"=w242:string)
                n127 = Concatenate Strings("cmd /c python createGdoc.py", w246, "KHZparameters.ini", w244, "KHZplaceholders.ini", w242, "KHZcurrentvalues.ini") -> (w240:string)
                n128 = property on="BASE PATH" class="Path"() -> ("Value"=w250:path)  [unwired: 2 in, 2 out]
                n129 = Build Path(base path=w250, name or relative path=path "GEECS-Plugins/LogMaker 4 GoogleDocs/source" ("working directory")) -> (appended path=w249:path)
                n130 = call <vilib>:"System Exec.vi"("expected output size  (4096)"=u32 1000000, "run minimized? (F)"=FALSE, "working directory"=w249, "command line"=w240) -> ()  [unwired: 4 in, 4 out]
              }
            }
            n131 = call <vilib>:"Add State(s) to Queue__jki_lib_state_machine.vi"("State(s) in (\"\")"=w237) -> ("States Out"=w238:string)  [unwired: 14 in]
          }
        }
      }
      frame "---------- Core ----------" {
        # "Do not put any code in this frame.\n(it is a separator no-op)"
        n132 = call <vilib>:"Add State(s) to Queue__jki_lib_state_machine.vi"("State(s) in (\"\")"=w256) -> ("States Out"=w255:string)  [unwired: 14 in]
      }
      frame Default {
        w266 = 42 items=["No error", "Argument error", "Memory is full", "Out of zone", "End of file", "File already open", "Generic file I/O error", "File not found", "File permission error", "Disk is full", "Duplicate path", "Too many files open", "System feature not enabled", "Resource file not found", "Cannot add resource", "Resource not found", "Image not found", "Image memory error", "Pen does not exist", "Config type invalid", "Config token not found", "Config parse error", "Config memory error", "Bad external code format", "Bad external code offset", "External code not present", "Null window", "Destroy window error", "Null menu", "Print aborted", "Bad print record", "Print driver error", "Windows error during printing", "Memory error during printing", "Print dialog error", "Generic print error", "Invalid device refnum", "Device not found", "Device parameter error", "Device unit error", "Cannot open device", "Device call aborted", "Generic error", "Cancelled by user", "Object ID too low", "Object ID too high", "Object not in heap", "Unknown heap", "Unknown object (invalid DefProc)", "Unknown object (DefProc not in table)", "Message out of range", "Invalid (null) method", "Unknown message", "Manager call not supported", "Bad address", "Network operation in progress", "Network operation timed out", "Connection is busy", "Network attribute not supported", "Network error", "Address in use", "System out of memory", "Connection aborted", "Connection refused", "Not connected", "Already connected", "Connection closed", "Initialization error (interapplication manager)", "Bad occurrence", "Wait on unbound occurrence handler", "Occurrence queue overflow", "Datalog type conflict", "Unused", "Unrecognized type (interapplication manager)", "Memory corrupt", "Failed to make temporary DLL", "Old CIN version", "Drag socket not found", "Failed to load drop-object", "Failed to register OLE object", "Failed to release OLE object", "Format specifier type mismatch", "Unknown format specifier", "Too few format specifiers", "Too many format specifiers", "Scan failed", "Newer CIN version", "Error converting to variant", "Runtime menu error", "Password tampered", "Variant attribute not found", "Incompatible variant data type", "Event data is not available", "Event Store is not present", "Occurrence is not found", "Event Queue is not created", "Event info is not available", "Refnum passed is NULL", "Error retrieving Class GUID", "Error retrieving CoClass GUID", "Error retrieving TypeLib GUID.", "Bad built application magic bytes.", "Specific driver is different from the specific driver associated with the Logical Name.", "There is no session opened to the class driver.", "Max Error", "MAX - Error with config objects", "MAX - Error loading configuration", "MAX - Group not supported"]
        # "Current State"
        # "Do not delete, rename, or modify this frame.\n(this is used to capture unhandled states and typos)"
        # "Handle mistyped state name (developer tool)"
        n133 = Format Into String(format string="Software Exception: Unhandled State \"%s\"." ("message"), error in=w262, w257) -> (resulting string=w265:string, error out=w264:errorcluster)  [unwired: 1 in]
        n134 = call <vilib>:"Error Cluster From Error Code.vi"("show call chain? (False)"=TRUE, "error in (no error)"=w264, "error message (\"\")"=w265, "error code (0)"=w266) -> ("error out"=w263:errorcluster)  [unwired: 5 in]
        n135 = call <vilib>:"Add State(s) to Queue__jki_lib_state_machine.vi"("State(s) in (\"\")"=w261) -> ("States Out"=w260:string)  [unwired: 14 in]
      }
      frame "Initialize Core Data" {
        # "Do not delete, rename, or modify this frame.\n(this is used to determine panel behavior on exit)"
        # "originally closed?"
        # "exe?"
        # "If panel starts closed or is an EXE, then close it when we exit"
        n136 = property class="VI"() -> ("FP.State"=w270:T7)  [unwired: 2 in, 2 out]
        n137 = property class="App"() -> ("App.Kind"=w276:T8)  [unwired: 2 in, 2 out]
        n138 = control-ref of="Current VI Reference"() -> (w271:refnum<vi>)
        n139 = Equal?(x=w270, y=T7."Closed" ("Front Panel Window:State")) -> (x = y?=w268:bool)
        n140 = Equal?(x=w276, y=T8."Run Time System" ("Application:Kind")) -> (x = y?=w274:bool)
        n141 = Or(x=w268, y=w274) -> (x .or. y?=w272:bool)
        n142 = Bundle By Name(cluster=w273, "Core.Current VI Reference"=w271, "Core.Close Panel on Exit?"=w272) -> (w278:T9)
        n143 = call <vilib>:"Add State(s) to Queue__jki_lib_state_machine.vi"("State(s) in (\"\")"=w280) -> ("States Out"=w279:string)  [unwired: 14 in]
      }
      frame "Error Handler" {
        # "Unhandled Error -- Display it"
        # "Handle any errors here.\nYou can also output any states to clean-up after errors occur"
        # "Clear error"
        n144 = call <vilib>:"General Error Handler.vi"("error in (no error)"=w282) -> ()  [unwired: 10 in, 5 out]
        n145 = call <vilib>:"Add State(s) to Queue__jki_lib_state_machine.vi"("State(s) in Front (\"\")"="/* Post Error States", "State(s) in (\"\")"=w286) -> ("States Out"=w285:string)  [unwired: 13 in]
      }
      frame "Exit" {
        # "Do not put any code in this frame.\n(No errors that occur here will be handled.)"
        n146 = call <vilib>:"Add State(s) to Queue__jki_lib_state_machine.vi"("State(s) in (\"\")"=w291) -> ("States Out"=w290:string)  [unwired: 14 in]
      }
      frame "---------- Data ----------" {
        # "Do not put any code in this frame.\n(It is a separator no-op. You can make a copy of this frame to create a new Data frame)"
        n147 = call <vilib>:"Add State(s) to Queue__jki_lib_state_machine.vi"("State(s) in (\"\")"=w295) -> ("States Out"=w294:string)  [unwired: 14 in]
      }
      frame "Data: Initialize" {
        w296 = FALSE  # ModeImagerIn
        w298 = FALSE  # Fire Continues Allowed
        w297 = u32 0  # Tik1
        w300 = FALSE  # Jet enable
        w299 = FALSE  # Jet trigger
        w301 = T12 {"Current VI Reference"=refnum, "Close Panel on Exit?"=FALSE}  # Core
        # "do not delete - used by framework"
        # "Expand Bundle to add new data elements to shift register data."
        # "Add new data here."
        # "Data names and types of shift register data are defined by this bundle."
        # "Initialize the shift-register data, here.\n(data names are defined by what you wire into the bundle function)"
        n148 = Bundle("Core"=w301, "Jet enable"=w300, "Jet trigger"=w299, "Fire Continues Allowed"=w298, "Tik1"=w297, "ModeImagerIn"=w296) -> (w303:T9)  [unwired: 1 in]
        n149 = call <vilib>:"Add State(s) to Queue__jki_lib_state_machine.vi"("State(s) in (\"\")"=w305) -> ("States Out"=w304:string)  [unwired: 14 in]
      }
      frame "Data: Cleanup" {
        # "Cleanup any data and references, here.\n(this is called automatically, by the Macro: Exit)"
        n150 = Unbundle By Name(w306) -> ("Core.Current VI Reference"=w309:refnum<vi>)
        n151 = Close Reference(reference=w309, error in (no error)=w308) -> (error out=w307:errorcluster)
        n152 = call <vilib>:"Add State(s) to Queue__jki_lib_state_machine.vi"("State(s) in (\"\")"=w311) -> ("States Out"=w310:string)  [unwired: 14 in]
      }
      frame "---------- UI ----------" {
        # "Do not put any code in this frame.\n(It is a separator no-op. You can make a copy of this frame to create a new UI frame)"
        n153 = call <vilib>:"Add State(s) to Queue__jki_lib_state_machine.vi"("State(s) in (\"\")"=w315) -> ("States Out"=w314:string)  [unwired: 14 in]
      }
      frame "UI: Initialize" {
        # "Initialize the User Interface, here.\n(this is called automatically, by the Macro: Init)"
        n154 = call <vilib>:"Add State(s) to Queue__jki_lib_state_machine.vi"("State(s) in (\"\")"=w319) -> ("States Out"=w318:string)  [unwired: 14 in]
      }
      frame "UI: Cursor Set" {
        # "Argument"
        # "Set and Unset Cursor Busy.\n(Usage: \"UI: Cursor Set >> Busy|Idle\")"
        n155 = case shown="\"Idle\", Default" w320 {
          tunnel: w322 -> [w327 w329]
          tunnel: [w326 w328] -> w321
          frame "Idle", Default {
            n156 = call <vilib>:"Unset Busy.vi"("error in (no error)"=w327) -> ("error out"=w326:errorcluster)  [unwired: 10 in]
          }
          frame "Busy" {
            n157 = call <vilib>:"Set Busy.vi"("error in (no error)"=w329) -> ("error out"=w328:errorcluster)  [unwired: 9 in, 1 out]
          }
        }
        n158 = call <vilib>:"Add State(s) to Queue__jki_lib_state_machine.vi"("State(s) in (\"\")"=w325) -> ("States Out"=w324:string)  [unwired: 14 in]
      }
      frame "UI: Front Panel State" {
        # "Argument"
        # "Set Front Panel Open or Closed\n(Usage: \"UI: Front Panel State >> Open|Close\")"
        n159 = Unbundle By Name(w332) -> ("Core.Current VI Reference"=w331:refnum<vi>)
        n160 = case shown="\"Minimize\", \"Minimized\"" w330 {
          tunnel: w334 -> [w342 w357 w368 w381 w394]
          tunnel: [w344 w358 w370 w383 w396] -> w333
          tunnel: w331 -> [w343 w355 w369 w382 w395]
          frame "Open", "Standard", Default {
            w337 = T7."Standard" ("State")
            n161 = property class="VI"(reference=w343, error in=w342) -> (reference out=w340:refnum<vi>, error out=w341:errorcluster, "FP.State"=w339:T7)
            n162 = Not Equal?(x=w339, y=w337) -> (x != y?=w338:bool)
            n163 = case shown="True" w338 {
              tunnel: [w348 w350] -> w344
              tunnel: w341 -> [w347 w350]
              tunnel: w340 -> [w346 _]
              tunnel: w337 -> [w345 _]
              frame True {
                n164 = invoke class="VI" method="FP.Open"(reference=w346, error in=w347, "Activate"=TRUE, "State"=w345) -> (error out=w348:errorcluster)  [unwired: 1 in, 4 out]
              }
              frame False {
              }
            }
          }
          frame "Close", "Closed" {
            n165 = property class="VI"(reference=w355, error in=w357) -> (reference out=w354:refnum<vi>, error out=w356:errorcluster, "FP.State"=w352:T7)
            n166 = Not Equal?(x=w352, y=T7."Closed" ("Front Panel Window:State")) -> (x != y?=w351:bool)
            n167 = case shown="True" w351 {
              tunnel: [w359 w362] -> w358
              tunnel: w356 -> [w359 w361]
              tunnel: w354 -> [_ w360]
              frame False {
              }
              frame True {
                n168 = invoke class="VI" method="FP.Close"(reference=w360, error in=w361) -> (error out=w362:errorcluster)  [unwired: 1 in, 2 out]
              }
            }
          }
          frame "Hidden", "Hide" {
            w363 = T7."Hidden" ("State")
            n169 = property class="VI"(reference=w369, error in=w368) -> (reference out=w366:refnum<vi>, error out=w367:errorcluster, "FP.State"=w365:T7)
            n170 = Not Equal?(x=w365, y=w363) -> (x != y?=w364:bool)
            n171 = case shown="True" w364 {
              tunnel: [w374 w375] -> w370
              tunnel: w367 -> [w373 w375]
              tunnel: w366 -> [w372 _]
              tunnel: w363 -> [w371 _]
              frame True {
                n172 = invoke class="VI" method="FP.Open"(reference=w372, error in=w373, "State"=w371) -> (error out=w374:errorcluster)  [unwired: 2 in, 4 out]
              }
              frame False {
              }
            }
          }
          frame "Minimize", "Minimized" {
            w376 = T7."Minimized" ("State")
            n173 = property class="VI"(reference=w382, error in=w381) -> (reference out=w379:refnum<vi>, error out=w380:errorcluster, "FP.State"=w378:T7)
            n174 = Not Equal?(x=w378, y=w376) -> (x != y?=w377:bool)
            n175 = case shown="True" w377 {
              tunnel: [w387 w388] -> w383
              tunnel: w380 -> [w386 w388]
              tunnel: w379 -> [w385 _]
              tunnel: w376 -> [w384 _]
              frame True {
                n176 = invoke class="VI" method="FP.Open"(reference=w385, error in=w386, "State"=w384) -> (error out=w387:errorcluster)  [unwired: 2 in, 4 out]
              }
              frame False {
              }
            }
          }
          frame "Maximize", "Maximized" {
            w389 = T7."Maximized" ("State")
            n177 = property class="VI"(reference=w395, error in=w394) -> (reference out=w392:refnum<vi>, error out=w393:errorcluster, "FP.State"=w391:T7)
            n178 = Not Equal?(x=w391, y=w389) -> (x != y?=w390:bool)
            n179 = case shown="True" w390 {
              tunnel: [w400 w401] -> w396
              tunnel: w393 -> [w399 w401]
              tunnel: w392 -> [w398 _]
              tunnel: w389 -> [w397 _]
              frame True {
                n180 = invoke class="VI" method="FP.Open"(reference=w398, error in=w399, "State"=w397) -> (error out=w400:errorcluster)  [unwired: 2 in, 4 out]
              }
              frame False {
              }
            }
          }
        }
        n181 = call <vilib>:"Add State(s) to Queue__jki_lib_state_machine.vi"("State(s) in (\"\")"=w336) -> ("States Out"=w335:string)  [unwired: 14 in]
      }
      frame "---------- Macro ----------" {
        # "Do not put any code in this frame.\n(It is a separator no-op. You can make a copy of this frame to create a new Macro frame)"
        n182 = call <vilib>:"Add State(s) to Queue__jki_lib_state_machine.vi"("State(s) in (\"\")"=w405) -> ("States Out"=w404:string)  [unwired: 14 in]
      }
      frame "Macro: Initialize" {
        w406 = "Data: Initialize\nInitialize Core Data\nUI: Initialize\nUI: Front Panel State >> Open"  # Data: Initialize Initialize Core Data UI: Initialize UI: Front Panel State >> Open
        # "Initialization Macro\n(This is called once, when the VI starts)"
        n183 = call <vilib>:"Add State(s) to Queue__jki_lib_state_machine.vi"("State(s) in Front (\"\")"=w406, "State(s) in (\"\")"=w410) -> ("States Out"=w409:string)  [unwired: 13 in]
      }
      frame "Macro: Exit" {
        # "Exit Macro\n(This is called once, when the VI exits)"
        n184 = Unbundle By Name(w417) -> ("Core.Close Panel on Exit?"=w416:bool)
        n185 = Select(t="UI: Front Panel State >> Close", s=w416, f="") -> (s? t:f=w413:string)
        n186 = call <vilib>:"Add State(s) to Queue__jki_lib_state_machine.vi"("State(s) in (\"\")"=w413, "State(s) at Back (\"\")"="Data: Cleanup\nExit") -> ("States Out"=w411:string)  [unwired: 13 in]
        n187 = call <vilib>:"Add State(s) to Queue__jki_lib_state_machine.vi"("State(s) in Front (\"\")"=w411, "State(s) in (\"\")"=w420) -> ("States Out"=w419:string)  [unwired: 13 in]
      }
      frame "---------- Action ----------" {
        # "Template Separator\n(You can make a copy of, or modify, this frame)"
        n188 = call <vilib>:"Add State(s) to Queue__jki_lib_state_machine.vi"("State(s) in (\"\")"=w424) -> ("States Out"=w423:string)  [unwired: 14 in]
      }
      frame "Action: Fire" {
        n189 = property on="fire::4" class="Str"(error in=w426, "Val(Sgnl)"="fire>>force" ("Value (Signaling)")) -> (error out=w425:errorcluster)  [unwired: 1 in, 1 out]
        n190 = call <vilib>:"Add State(s) to Queue__jki_lib_state_machine.vi"("State(s) in (\"\")"=w430) -> ("States Out"=w429:string)  [unwired: 14 in]
      }
      frame "Action: template" {
        n191 = call <vilib>:"Add State(s) to Queue__jki_lib_state_machine.vi"("State(s) in (\"\")"=w434) -> ("States Out"=w433:string)  [unwired: 14 in]
      }
      frame "Initilize Fire Continues" {
        n192 = Unbundle By Name(w437) -> ("Fire Continues Allowed"=w439:bool)
        n193 = property on="value0:6" class="Bool (strict)"(error in=w436, "Visible"=w439) -> (error out=w440:errorcluster)  [unwired: 1 in, 1 out]
        n194 = Not(x=w439) -> (.not. x?=w438:bool)
        n195 = property on="Fire continues Indicator" class="Bool (strict)"(error in=w440, "Visible"=w438) -> (error out=w435:errorcluster)  [unwired: 1 in, 1 out]
        n196 = call <vilib>:"Add State(s) to Queue__jki_lib_state_machine.vi"("State(s) in (\"\")"=w442) -> ("States Out"=w441:string)  [unwired: 14 in]
      }
      frame "Action: Check if Fire continues cllowed" {
        # "Check if it is allowed computer"
        # "Template Separator\n(You can make a copy of, or modify, this frame)"
        n197 = String To IP() -> (0:w450:u32)  [unwired: 1 in]
        n198 = IP To String(1:TRUE ("dot notation? (F)"), 2:w450) -> (0:w451:string)
        n199 = Equal?(x=w451, y="192.168.7.228") -> (x = y?=w447:bool)
        n200 = Not(x=w447) -> (.not. x?=w448:bool)
        n201 = Bundle By Name(cluster=w446, "Fire Continues Allowed"=w447) -> (w445:T9)
        n202 = property on="Fire Continues Checkbox" class="Bool (strict)"(error in=w443, "Visible"=w448) -> (error out=w444:errorcluster)  [unwired: 1 in, 1 out]
        n203 = call <vilib>:"Add State(s) to Queue__jki_lib_state_machine.vi"("State(s) in (\"\")"=w454) -> ("States Out"=w453:string)  [unwired: 14 in]
      }
      frame "Action: CheckTimeFire" {
        # "Your code here.\n(You can make a copy of, or modify, this frame)"
        n204 = Unbundle By Name(w458) -> ("Tik1"=w464:u32)
        n205 = Tick Count (ms)() -> (millisecond timer value=w462:u32)
        n206 = Unbundle By Name(w458) -> ("Fire Continues Allowed"=w468:bool)
        n207 = Reciprocal(x="Rate (Hz)") -> (1/x=w469:dbl)
        n208 = Subtract(x=w462, y=w464) -> (x-y=w461:u32)
        n209 = Multiply(x=1000.0, y=w469) -> (x*y=w470:dbl)
        n210 = Greater?(x=w461, y=w470) -> (0:w465:bool)
        n211 = And(x=w465, y="value0:6") -> (x .and. y?=w466:bool)
        n212 = And(x=w468, y=w466) -> (x .and. y?=w467:bool)
        n213 = case shown="True" w467 {
          tunnel: w462 -> [_ w476]
          tunnel: [w474 w476] -> w463
          tunnel: w464 -> [w474 _]
          tunnel: [_ "Action: Fire" ("State(s) in Front (\"\")")] -> w459
          frame False {
          }
          frame True {
          }
        }
        n214 = Bundle By Name(cluster=w458, "Tik1"=w463) -> (w457:T9)
        n215 = call <vilib>:"Add State(s) to Queue__jki_lib_state_machine.vi"("State(s) in Front (\"\")"=w459, "State(s) in (\"\")"=w473) -> ("States Out"=w472:string)  [unwired: 13 in]
        "Fire continues Indicator" <- "value0:6"
      }
    }
  }
